vi "FTW-TestStep-Base_ReportResults.vi"(0 "FTW-TestStep-Base In":refnum<class "FTW-TestStep-Base.lvclass">, 5 "Passed":bool, 7 "Additional Results":variant, 11 "error in (no error)":errorcluster) -> (4 "FTW-TestStep-Base Out":refnum<class "FTW-TestStep-Base.lvclass">, 15 "error out":errorcluster)   [LabVIEW 2018, in "FTW-TestStep-Base.lvclass"]
uses:
  FTW-TestStep-Base.lvclass
  TestExecutive/FTW-TestExecutive-Results.ctl
  FTW-TestStep-Base.lvclass/FTW-TestStep-Base.ctl
  Connector/FTW-ActorConnector.lvclass
  125fa722-c9f1-42e7-9d6f-45884d3376a1.vi
  125fa722-c9f1-42e7-9d6f-45884d3376a1.vi/2e34f099-65ab-491b-9a22-30028d269259.vi
  container/FTW-Container-FromVariant.vi
  container/FTW-Container-New-FromContainer.vi
  JSON/FTW-JSON-SerializeAndDestroy.vi
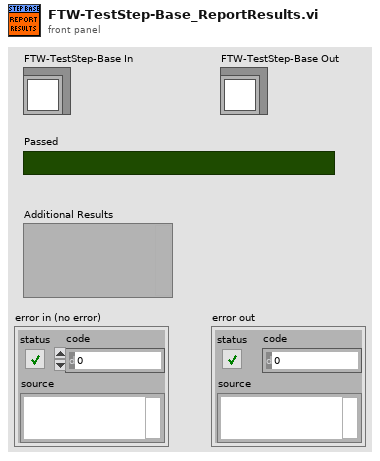
[diagram p1: front panel]
types:
  T1 = typedef "FTW-TestExecutive-Results.ctl" = cluster{"Start Time":timestamp, "Elapsed Time":dbl, "Passed":bool, "Additional Results":string}
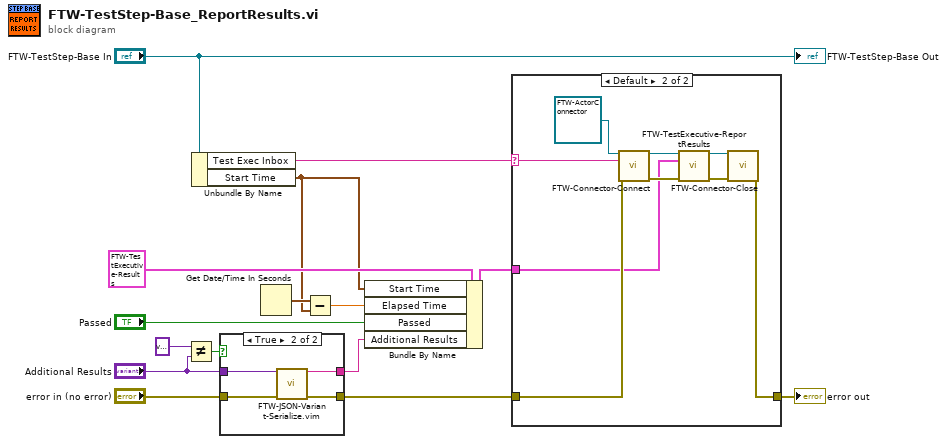
[diagram p0: block diagram]
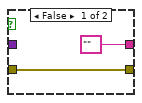
[diagram p2: hidden frame]
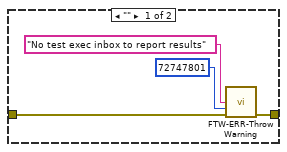
[diagram p3: hidden frame]
diagram:
  n1 = Not Equal?(x=variant, y="Additional Results") -> (x != y?=w4:bool)
  n2 = Unbundle By Name("FTW-TestStep-Base In") -> ("Test Exec Inbox"=w9:string, "Start Time"=w1:timestamp)
  n3 = case shown="True" w4 {
    tunnel: "error in (no error)" -> [w16 w21]
    tunnel: [w16 w20] -> w6
    tunnel: "Additional Results" -> [_ w19]
    tunnel: ["" ("empty string") w18] -> w2
    frame False {
    }
    frame True {
      n4 = call "FTW-JSON-Variant-Serialize.vim"("Variant"=w19, "error in"=w21) -> ("JSON String"=w18:string, "error out"=w20:errorcluster)  [unwired: 12 in]
    }
  }
  n5 = Get Date/Time In Seconds() -> (seconds since 1Jan1904=w8:timestamp)
  n6 = Subtract(x=w8, y=w1) -> (x-y=w7:dbl)
  n7 = Bundle By Name(cluster=T1 {"Start Time"=timestamp(0 s since 1904-01-01), "Elapsed Time"=0.0, "Passed"=FALSE, "Additional Results"=""} ("Results"), "Start Time"=w1, "Elapsed Time"=w7, "Passed"="Passed", "Additional Results"=w2) -> (w12:T1)
  n8 = case shown="Default" w9 {
    selector: w9 -> [_ w26]
    tunnel: [w24 w31] -> w15
    tunnel: w6 -> [w25 w28]
    tunnel: w12 -> [_ w27]
    frame "" {
      n9 = call "FTW-ERR-ThrowWarning.vi"("Warning Message"="No test exec inbox to report results" ("Error Message"), "Error Code"=72747801, "error in"=w25) -> ("error out"=w24:errorcluster)  [unwired: 12 in]
    }
    frame Default {
      n10 = call-dynamic "FTW-Connector-Connect.vi"("FTW Actor Connector Type"=refnum<class "FTW-ActorConnector.lvclass"> refnum, "Instance Inbox Address"=w26, "error in"=w28) -> ("FTW Actor Connector"=w33:refnum<class "FTW-ActorConnector.lvclass">, "error out"=w29:errorcluster)  [unwired: 11 in]
      n11 = call "FTW-TestExecutive-ReportResults.vi"("FTW Actor Connector In"=w33, "Results"=w27, "error in (no error)"=w29) -> ("FTW Actor Connector"=w34:refnum<class "FTW-ActorConnector.lvclass">, "error out"=w32:errorcluster)  [unwired: 9 in, 2 out]
      n12 = call-dynamic "FTW-Connector-Close.vi"("FTW Actor Connector"=w34, "error in"=w32) -> ("error out"=w31:errorcluster)  [unwired: 13 in]
    }
  }
  "error out" <- w15
  "FTW-TestStep-Base Out" <- "FTW-TestStep-Base In"
